vi "Mass Rename Window Titles.vi"() -> ()   [LabVIEW 2020]
panel:
  out "error out":errorcluster
  out "VIs Total":i32
  out "VIs Processed":i32
  in  "Replace String":string
  in  "Search String":string
  in  "Folder":path
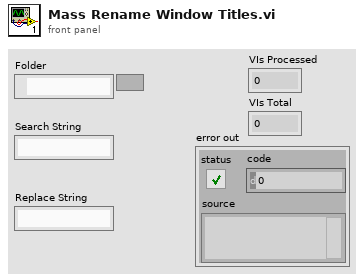
[diagram p1: front panel]
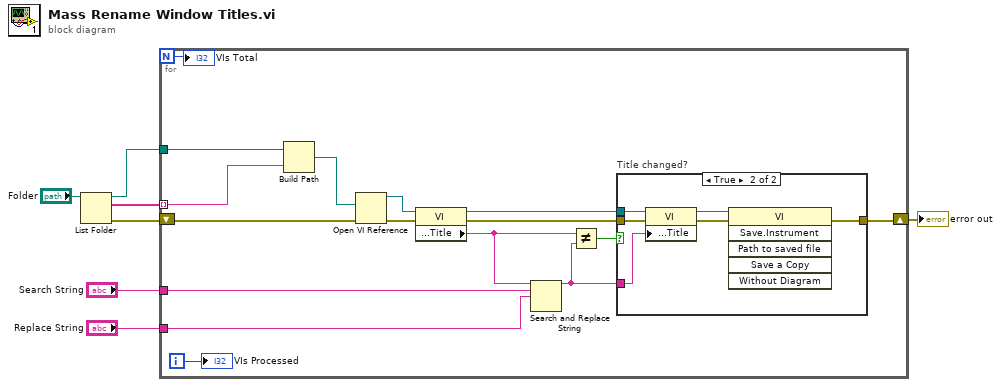
[diagram p0: block diagram]
diagram:
  n1 = List Folder(path="Folder") -> (path out=w5:path, filenames=w6:string[], error out=w4:errorcluster)  [unwired: 3 in, 1 out]
  n2 = for {
    N -> [w8]
    tunnel: w6 -> [w22] mode=indexing
    tunnel: w5 -> [w23]
    tunnel: "Search String" -> [w17]
    tunnel: "Replace String" -> [w16]
    shift-right: [w13] -> w1
    shift-left: w4 -> [w21]
    i -> [w9]
    n3 = Build Path(base path=w23, name or relative path=w22) -> (appended path=w20:path)
    n4 = Open VI Reference(vi path=w20, error in (no error)=w21) -> (vi reference=w19:refnum<vi>, error out=w15:errorcluster)  [unwired: 4 in]
    n5 = property class="VI"(reference=w19, error in=w15) -> (reference out=w18:refnum<vi>, error out=w14:errorcluster, "Front Panel.Title"=w11:string)
    n6 = Search and Replace String(input string=w11, search string=w17, replace string=w16) -> (result string=w12:string)  [unwired: 5 in, 3 out]
    n7 = Not Equal?(x=w11, y=w12) -> (x != y?=w10:bool)
    n8 = case "Title changed?" shown="True" w10 {
      tunnel: w18 -> [_ w30]
      tunnel: w14 -> [w24 w28]
      tunnel: [w24 w26] -> w13
      tunnel: w12 -> [_ w25]
      frame False {
      }
      frame True {
        n9 = property class="VI"(reference=w30, error in=w28, "Front Panel.Title"=w25) -> (reference out=w29:refnum<vi>, error out=w27:errorcluster)
        n10 = invoke class="VI" method="Save.Instrument"(reference=w29, error in=w27) -> (error out=w26:errorcluster)  [unwired: 4 in, 5 out]
      }
    }
    "VIs Processed" <- w9
    "VIs Total" <- w8
  }
  "error out" <- w1
